vi "CALC_Mouse_angular_position_in_the_cage's_coordinates.vi"(1 "abs(theta) < pi, rad":dbl[](array[numeric]), 2 "a, rad":dbl[](array[numeric])) -> (0 "phi, rad":dbl[](array[numeric]))   [LabVIEW 2018, in "Tracker.lvlib"]
uses:
  Tracker.lvlib
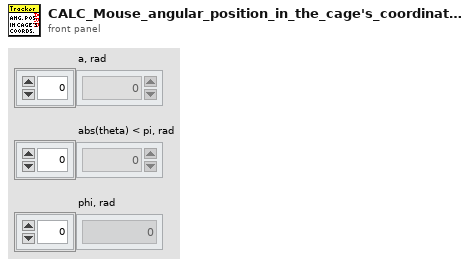
[diagram p1: front panel]
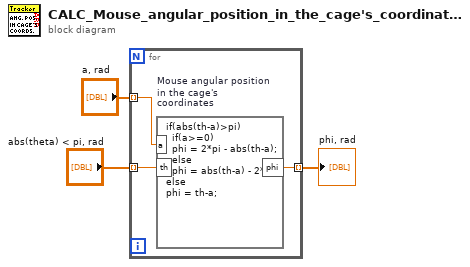
[diagram p0: block diagram]
diagram:
  n1 = for {
    tunnel: "abs(theta) < pi, rad" -> [w6] mode=indexing
    tunnel: [w5] -> w1 mode=indexing
    tunnel: "a, rad" -> [w4] mode=indexing
    n2 = formula code="if(abs(th-a)>pi)\n  if(a>=0)\n  phi = 2*pi - abs(th-a);\n  else\n  phi = abs(th-a) - 2*pi;\nelse\nphi = th-a;" "Mouse angular position in the cage's coordinates"("th"=w6, "a"=w4) -> ("phi"=w5:dbl)
  }
  "phi, rad" <- w1
